vi "final_usrp_transceiver.vi"() -> ()   [LabVIEW 2014]
uses:
  <vilib>/vision/Image Controls.llb/IMAQ Image.ctl
  <vilib>/addons/Modulation/Digital/General/MT Generate Bits (Galois, PN Order).vi
  <vilib>/Analysis/2dsp.llb/Inverse Complex FFT.vi
  <vilib>/Analysis/2dsp.llb/Complex FFT.vi
  <vilib>/Analysis/5stat.llb/RMS (DBL).vi
  <vilib>/addons/Modulation/Digital/Support/Common/Validators/mod_Generate Bits Validate.vi
  <vilib>/addons/Modulation/Analog/support/mod_Set Error Source.vi
  var_stop.vi
  <vilib>/addons/Modulation/Digital/Support/Common/Validators/mod_Generate Filter Coefficients Validate.vi
  <vilib>/addons/Modulation/Digital/General/subVIs/mod_Generate Filter Coefficients.vi
  <vilib>/addons/Modulation/Digital/General/subVIs/mod_Generate Bits PN Sequence.vi
  <vilib>/addons/Modulation/Digital/General/MT Generate QAM System Parameters(M).vi
  <vilib>/addons/Modulation/Digital/General/MT Apply Pulse Shaping Filter (Generic).vi
  <instrlib>/niUSRP/niUSRP Write Tx Data (CDB Cluster).vi
  <vilib>/addons/Modulation/Digital/General/MT Apply Matched Filter (Generic).vi
  <vilib>/addons/Modulation/Digital/General/MT Align to Ideal Symbols (Generic).vi
  <vilib>/addons/Modulation/Digital/General/MT Map QAM Symbols to Bits.vi
  <instrlib>/niUSRP/niUSRP Fetch Rx Data (CDB Cluster).vi
  <vilib>/addons/Modulation/niDMT.lvlib
  <vilib>/Analysis/NI_AALPro.lvlib
panel:
  out "frame":T1(plugin-control)
  out "length 2":i32
  out "string":string
  out "number":u32
  out "pilot channel gain":dbl[](graph)
  out "pilot channel gain":dbl[](graph)
  out "PAPR":dbl
  in  "M-QAM (16)":i32=16
  out "TX buffer":i32
  out "RX buffer":i32
  out "avg energy":dbl
  in  "TX on":bool=TRUE
  in  "power scale":dbl format="%#_13g"
  out "acc recieved bits":i32
  out "acc error bits":i32
  out "Packet number":u8
  out "Packet bytes":u32
  out "past 20 error bits":i32[](array[numeric])
  in  "min_len":i32=200
  in  "Threshold":dbl=-61.0 format="%#_13g"
  out "Accumulated BER":dbl
  out "found packet":bool
  in  "total bits (128)":i32=1600 caption="bits per packet"
  in  "message carriers":i32=120
  out "RX  constellation map":cdb[](graph)
  in  "pilot carrier":i32=32
  in  "cyclic length":i32=64
  in  "FFT size":i32=256
  in  "filter length (symbols)":i32=8
  in  "filter parameter":dbl=0.35 format="%.2f"
  in  "samples per symbol (16)":i32=4
  in  "pulse shaping filter (none)":T2(ring)=enum."Root Raised Cos"
  in  "stop":bool
  in  "number of samples":i64=20000
  out "coerced carrier frequency":dbl format="%#_6p"
  out "coerced IQ rate":dbl format="%#_6p"
  in  "Clocking and Synchronization:Reference Frequency Source":string(combo)="Internal"
  in  "RX gain":dbl format="%#_6f"
  in  "TX gain":dbl format="%#_6f"
  in  "carrier frequency":dbl=915000000.0 format="%#_6p"
  in  "IQ rate":dbl=2000000.0 format="%#_6p"
  in  "RX device names":refnum<k15>="192.168.10.3"
  in  "TX device names":refnum<k15>="192.168.10.3"
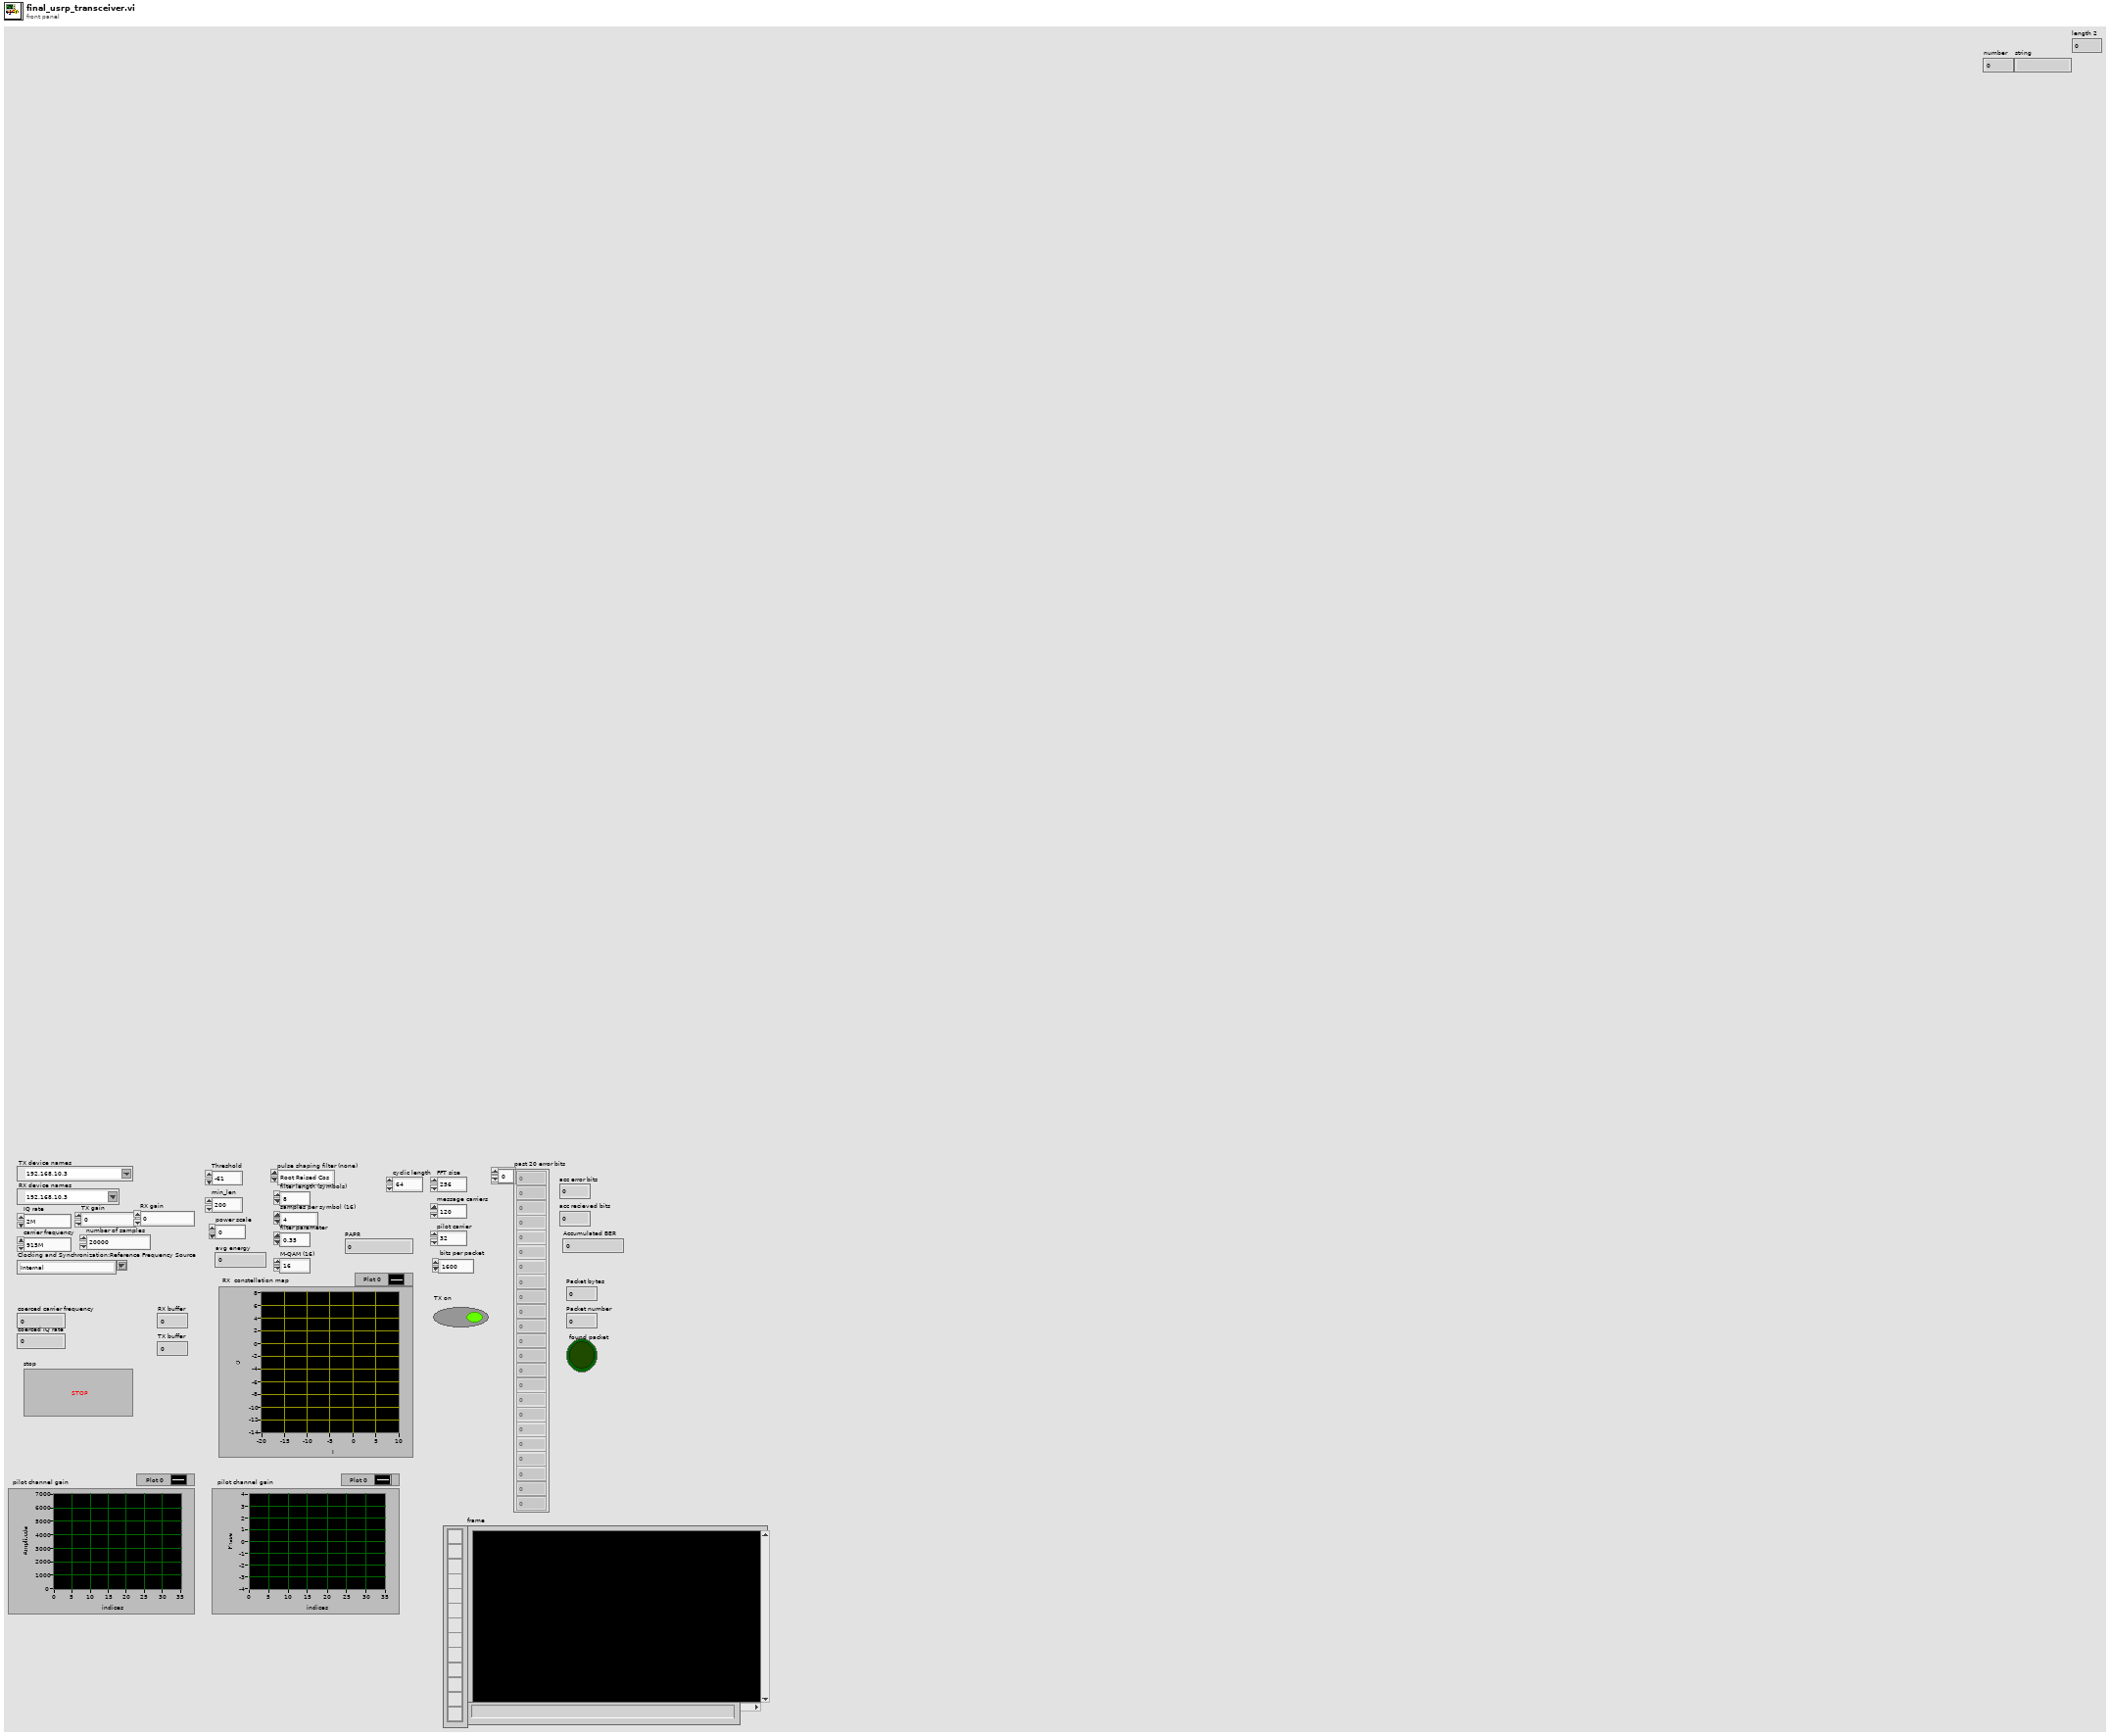
[diagram p1: front panel]
types:
  T1 = typedef "IMAQ Image.ctl" = refnum<image>
  T2 = enum16{"none", "Raised Cosine", "Root Raised Cos", "Gaussian"}
  T3 = enum16{"FSK", "PSK", "QAM", "MSK", "PAM", "ASK", "CPM"}
  T4 = cluster{"samples per symbol (16)":i32, "symbol map":cdb[]}
  T5 = typedef "niAMT.lvlib/Complex Data Waveform.ctl" = cluster{"t0":dbl, "dt":dbl, "Y":cdb[]}
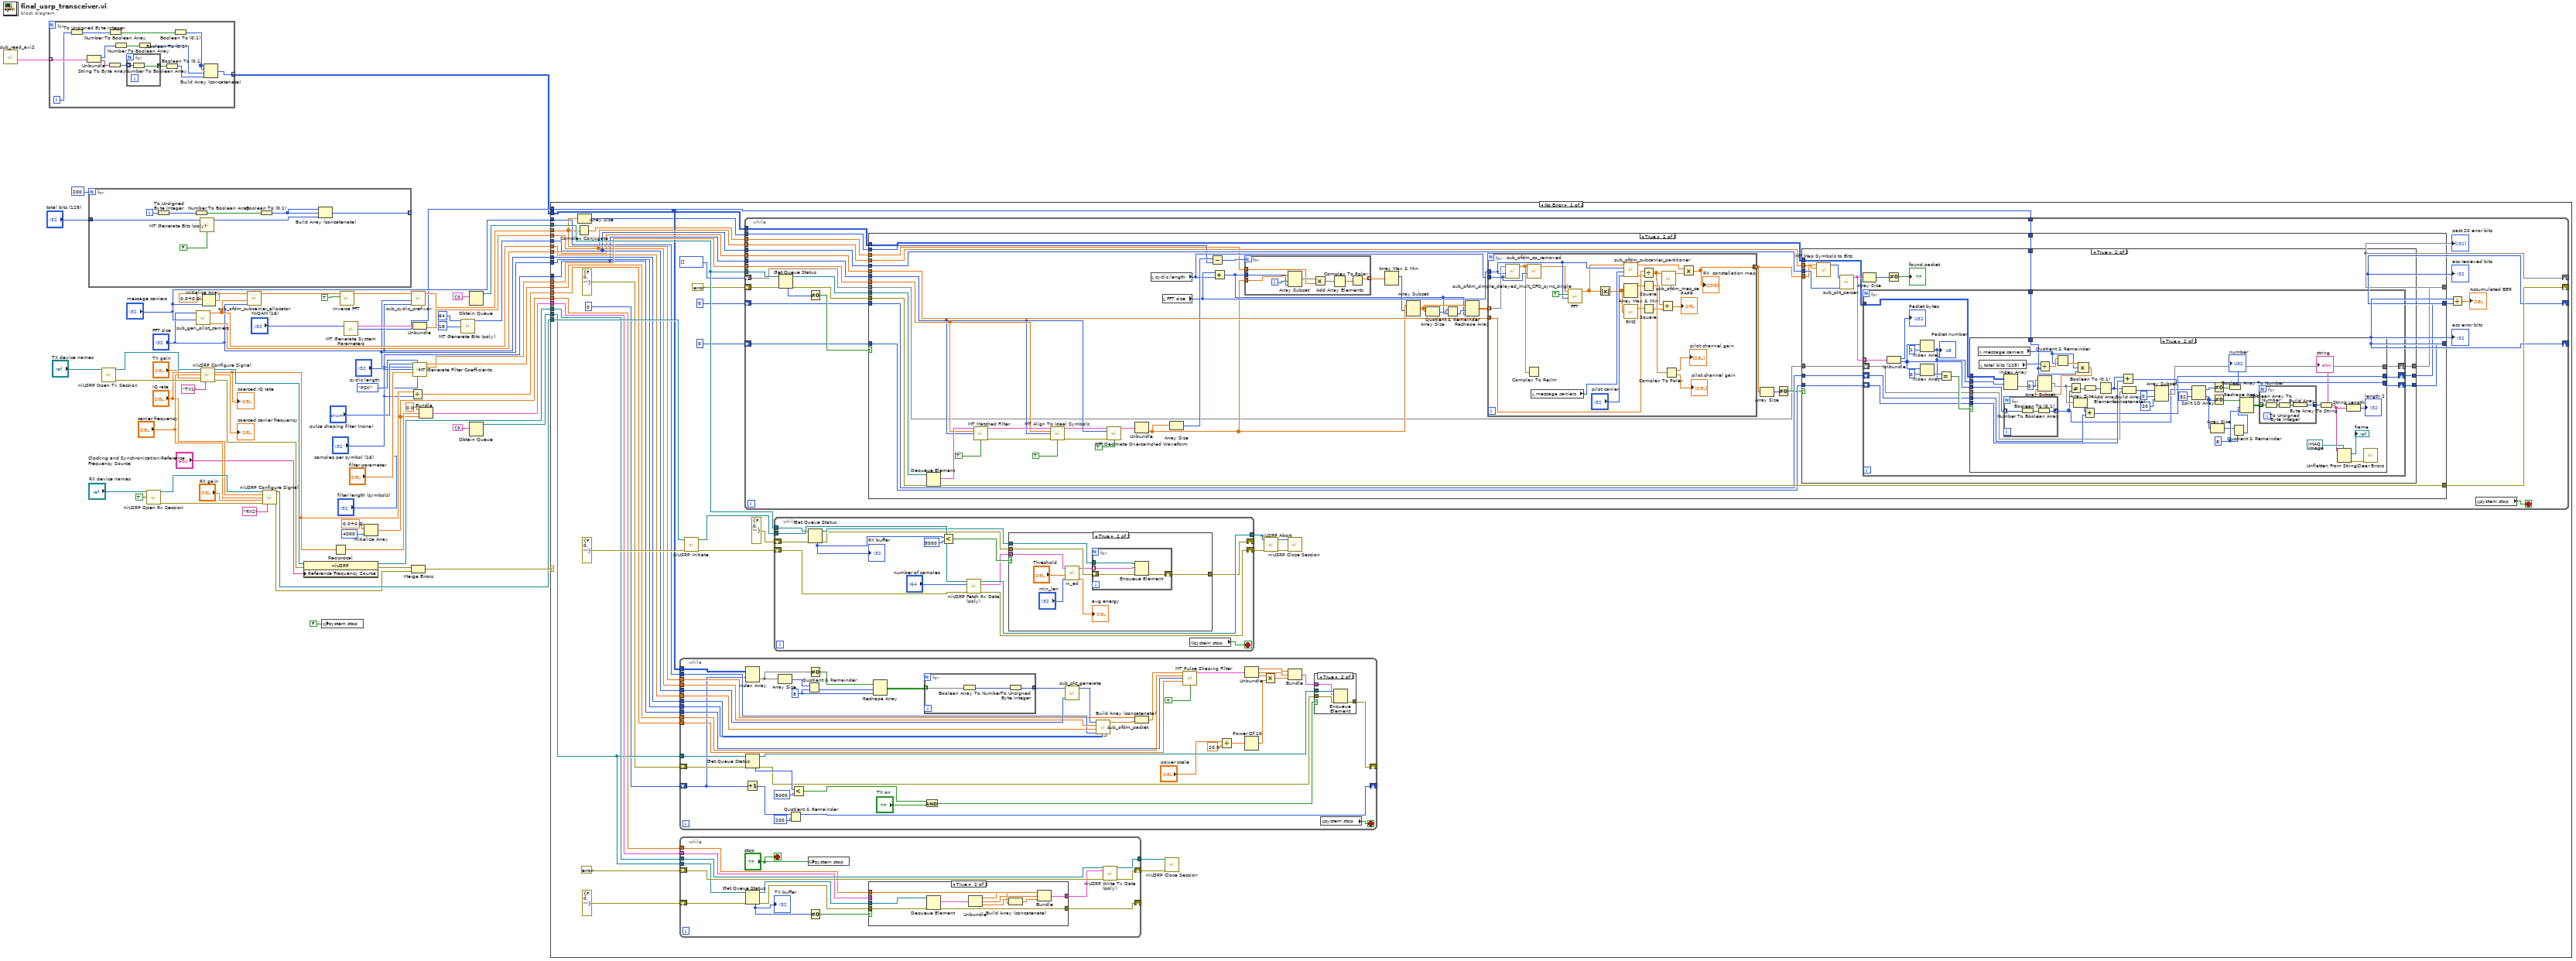
[diagram p0: block diagram]
diagram:
  n1 = call "sub_read_avi2.vi"() -> ("frames"=w2:cluster{i32, "Data String":string}[])  [unwired: 10 in, 1 out]
  n2 = for {
    tunnel: w2 -> [w70] mode=indexing
    tunnel: [w69] -> w1 mode=indexing
    i -> [w66]
    n3 = To Unsigned Byte Integer(number=w66) -> (unsigned 8bit integer=w68:u8)
    n4 = Unbundle(w70) -> (w75:i32, "Data String"=w71:string)
    n5 = String To Byte Array(string=w71) -> (unsigned byte array=w77:u8[])
    n6 = Number To Boolean Array(number=w68) -> (Boolean array=w67:bool[])
    n7 = Number To Boolean Array(number=w75) -> (Boolean array=w74:bool[])
    n8 = for {
      tunnel: w77 -> [w79] mode=indexing
      tunnel: [w78] -> w76 mode=concatenating
      n9 = Number To Boolean Array(number=w79) -> (Boolean array=w78:bool[])
    }
    n10 = Boolean To (0,1)(Boolean=w74) -> (0, 1=w72:i16[])
    n11 = Boolean To (0,1)(Boolean=w76) -> (0, 1=w73:i16[])
    n12 = Boolean To (0,1)(Boolean=w67) -> (0, 1=w65:i16[])
    n13 = Build Array (concatenate)(w65, w65, w72, w73) -> (w69:i16[])
  }
  n14 = for {
    N: 200 ("y") -> [_]
    tunnel: "total bits (128)" -> [w87]
    tunnel: [w80] -> _ mode=indexing
    i -> [w85]
    n15 = To Unsigned Byte Integer(number=w85) -> (unsigned 8bit integer=w84:u8)
    n16 = Number To Boolean Array(number=w84) -> (Boolean array=w83:bool[])
    n17 = call-poly <vilib>:"MT Generate Bits (poly).vi"("total bits (128)"=w87, "reset? (T)"=FALSE) -> ("output bit stream"=w81:i8[])  [unwired: 11 in, 2 out]
    n18 = Boolean To (0,1)(Boolean=w83) -> (0, 1=w82:i16[])
    n19 = Build Array (concatenate)(w82, w82, w81) -> (w80:i16[])
  }
  n20 = call <instrlib>:"niUSRP Open Tx Session.vi"("device names"="TX device names") -> ("session handle out"=w64:refnum<k15>, "error out"=w63:errorcluster)  [unwired: 13 in]
  n21 = call <instrlib>:"niUSRP Open Rx Session.vi"("device names"="RX device names", "reset"=TRUE) -> ("session handle out"=w60:refnum<k15>, "error out"=w59:errorcluster)  [unwired: 12 in]
  n22 = call "sub_gen_pilot_carriers.vi"("message carrier"="message carriers", "FFT size"="FFT size") -> ("RX pilot carriers"=w21:cdb[], "TX pilot carriers"=w17:cdb[])  [unwired: 8 in]
  n23 = call <instrlib>:"niUSRP Configure Signal.vi"("session handle"=w64, "IQ rate"="IQ rate", "carrier frequency"="carrier frequency", "gain"="TX gain", "error in (no error)"=w63, "active antenna"="TX1") -> ("session handle out"=w31:refnum<k15>, "coerced IQ rate"=w20:dbl, "coerced carrier frequency"=→"coerced carrier frequency":dbl, "error out"=w30:errorcluster)  [unwired: 5 in, 1 out]
  "coerced IQ rate" <- w20
  n24 = Initialize Array(cdb 0.0+0.0i, "message carriers") -> (w23:cdb[])
  n25 = call "sub_ofdm_subcarrier_allocator.vi"("fft size"="FFT size", "pilot symbol"=w17, "message symbol"=w23) -> ("OFDM symbol"=w16:cdb[])  [unwired: 8 in]
  n26 = call <instrlib>:"niUSRP Configure Signal.vi"("session handle"=w60, "IQ rate"="IQ rate", "carrier frequency"="carrier frequency", "gain"="RX gain", "error in (no error)"=w59, "active antenna"="RX2") -> ("session handle out"=w4:refnum<k15>, "error out"=w3:errorcluster)  [unwired: 5 in, 3 out]
  n27 = property class="niUSRP"(reference=w31, error in=w30, "Reference Frequency Source"="Clocking and Synchronization:Reference Frequency Source") -> (reference out=w45:refnum<k15>, error out=w50:errorcluster)
  n28 = global write "var_stop.vi" "system stop"(FALSE) -> ()
  n29 = Reciprocal(x=w20) -> (1/x=w40:dbl)
  n30 = call-poly <vilib>:"Inverse FFT.vi"("shift?"=TRUE, "FFT {X}"=w16) -> ("X"=w14:cdb[])  [unwired: 8 in, 1 out]
  n31 = call-poly <vilib>:"MT Generate System Parameters.vi"("M-QAM (16)"="M-QAM (16)") -> ("QAM system parameters"=w29:T4, "bits per symbol"=w6:i32)  [unwired: 12 in, 1 out]
  n32 = Initialize Array(cdb 0.0+0.0i, 4000 ("dimension size")) -> (w8:cdb[])
  n33 = Divide(x=w20, y="samples per symbol (16)") -> (x/y=w19:dbl)
  n34 = call "sub_cyclic_prefixer.vi"("FFT size"="FFT size", "CP length"="cyclic length", "time_samples"=w14) -> ("cp ofdm symbol"=w11:cdb[])  [unwired: 8 in]
  n35 = Merge Errors(w50, w3) -> (w49:errorcluster)
  n36 = Unbundle(w29) -> ("symbol map"=w28:cdb[])  [unwired: 1 out]
  n37 = call <vilib>:"MT Generate Filter Coefficients.vi"("pulse shaping filter (none)"="pulse shaping filter (none)", "modulation type"=T3."PSK", "pulse shaping samples per symbol (16)"="samples per symbol (16)", "matched samples per symbol (16)"="samples per symbol (16)", "filter parameter"="filter parameter", "filter length (symbols)"="filter length (symbols)") -> ("pulse shaping filter coefficients"=w34:dbl[], "matched filter coefficients"=w33:dbl[])  [unwired: 7 in, 1 out]
  n38 = Bundle(0.0, w40, w8) -> (w38:cluster{dbl, dbl, cdb[]})  [unwired: 1 in]
  n39 = call-poly <vilib>:"MT Generate Bits (poly).vi"("total bits (128)"=64, "PN sequence order (9)"=15) -> ("output bit stream"=w25:i8[])  [unwired: 11 in, 2 out]
  n40 = Obtain Queue(element data type=cluster{"t0":dbl, "dt":dbl, "Y":cdb[]} {"t0"=0.0, "dt"=0.0, "Y"=[]} ("data")) -> (queue out=w46:refnum<queue>)  [unwired: 4 in, 2 out]
  n41 = Obtain Queue(element data type=cluster{"t0":dbl, "dt":dbl, "Y":cdb[]} {"t0"=0.0, "dt"=0.0, "Y"=[]} ("data")) -> (queue out=w43:refnum<queue>)  [unwired: 4 in, 2 out]
  n42 = case shown="No Error" w49 {
    tunnel: w4 -> [w125 _]
    tunnel: w46 -> [w120 _]
    tunnel: w45 -> [w115 _]
    tunnel: w43 -> [w112 _]
    tunnel: w38 -> [w113 _]
    tunnel: w34 -> [w110 _]
    tunnel: w33 -> [w109 _]
    tunnel: "message carriers" -> [w106 _]
    tunnel: "FFT size" -> [w105 _]
    tunnel: w28 -> [w104 _]
    tunnel: w25 -> [w103 _]
    tunnel: w21 -> [w102 _]
    tunnel: w19 -> [w101 _]
    tunnel: "samples per symbol (16)" -> [w98 _]
    tunnel: w17 -> [w100 _]
    tunnel: "cyclic length" -> [w99 _]
    tunnel: w11 -> [w92 _]
    tunnel: w1 -> [w96 _]
    tunnel: w8 -> [w93 _]
    tunnel: w6 -> [w88 _]
    frame No Error {
      n43 = Complex Conjugate(1:w92) -> (0:w90:cdb[])
      n44 = Array Size(array=w92) -> (size(s)=w91:i32)
      n45 = while {
        tunnel: w112 -> [w167]
        shift-right: [w169] -> _
        shift-left: errorcluster {"status"=FALSE, "code"=0, "source"=""} ("error out") -> [w168]
        tunnel: w100 -> [w159]
        tunnel: w110 -> [w166]
        tunnel: w98 -> [w165]
        tunnel: w101 -> [w164]
        tunnel: w106 -> [w158]
        tunnel: w105 -> [w157]
        tunnel: w104 -> [w160]
        tunnel: w103 -> [w162]
        tunnel: w99 -> [w156]
        tunnel: w92 -> [w155]
        tunnel: w96 -> [w152]
        shift-right: [w148] -> _
        shift-left: 0 -> [w151]
        stop <- w174 stop-if-true
        w145 = 8 ("y")
        n46 = Increment(x=w151) -> (x+1=w150:i32)
        n47 = Index Array(array=w152, index (row)=w151) -> (element=w144:i16[])  [unwired: 1 in]
        n48 = Get Queue Status(queue=w167, error in (no error)=w168) -> (queue out=w171:refnum<queue>, error out=w170:errorcluster, # elements in queue=w173:i32)  [unwired: 1 in, 5 out]
        n49 = Array Size(array=w144) -> (size(s)=w147:i32)
        n50 = Quotient & Remainder(x=w150, y=200) -> (x-y*floor(x/y)=w148:i32)  [unwired: 1 out]
        n51 = Less?(x=w173, y=5000) -> (x < y?=w130:bool)
        n52 = Quotient & Remainder(x=w147, y=w145) -> (floor(x/y)=w146:i32)  [unwired: 1 out]
        n53 = Not Equal To 0?(x=w144) -> (x != 0?=w143:bool[])
        n54 = Reshape Array(w143, w146, w145) -> (w142:bool[][])
        n55 = for {
          tunnel: w142 -> [w177] mode=indexing
          tunnel: [w175] -> w141 mode=indexing
          n56 = Boolean Array To Number(Boolean array=w177) -> (number=w176:u32)
          n57 = To Unsigned Byte Integer(number=w176) -> (unsigned 8bit integer=w175:u8)
        }
        n58 = And(x=w130, y="TX on") -> (x .and. y?=w128:bool)
        n59 = call "sub_pkt_generate.vi"("accesscode (bit)"=w162, "byte stream"=w141) -> ("bit pkt"=w161:i16[])  [unwired: 9 in]
        n60 = call "sub_ofdm_packet.vi"("CP length"=w156, "FFT size"=w157, "message carriers"=w158, "pilot symbol"=w159, "symbol map"=w160, "packet"=w161) -> ("ofdm packet"=w154:cdb[])  [unwired: 5 in]
        n61 = Build Array (concatenate)(w155, w154) -> (w153:cdb[])
        n62 = call-poly <vilib>:"MT Pulse Shaping Filter.vi"("symbols"=w153, "pulse shaping filter coefficients"=w166, "samples per symbol (16)"=w165, "symbol rate (Hz)"=w164, "reset? (T)"=TRUE) -> ("output complex waveform"=w137:T5)  [unwired: 9 in, 1 out]
        n63 = Divide(x="power scale", y=20.0) -> (x/y=w138:dbl)
        n64 = Unbundle(w137) -> ("t0"=w132:dbl, "dt"=w133:dbl, "Y"=w136:cdb[])
        n65 = Power Of 10(x=w138) -> (10^x=w135:dbl)
        n66 = Multiply(x=w136, y=w135) -> (x*y=w134:cdb[])
        n67 = Bundle("t0"=w132, "dt"=w133, w134) -> (w131:cluster{"t0":dbl, "dt":dbl, cdb[]})  [unwired: 1 in]
        n68 = case shown="True" w128 {
          tunnel: w171 -> [_ w182]
          tunnel: w170 -> [w178 w181]
          tunnel: [w178 w180] -> w169
          tunnel: w131 -> [_ w179]
          frame False {
          }
          frame True {
            n69 = Enqueue Element(queue=w182, element=w179, error in (no error)=w181) -> (error out=w180:errorcluster)  [unwired: 1 in, 2 out]
          }
        }
        n70 = global read "var_stop.vi" "system stop"() -> (w174:bool)
      }
      n71 = while {
        tunnel: [w411] -> w118
        shift-right: [w410] -> w117
        shift-left: errorcluster {"status"=FALSE, "code"=0, "source"=""} ("error out") -> [w408]
        tunnel: w115 -> [w409]
        tunnel: w112 -> [w407]
        shift-right: [w401] -> _
        shift-left: errorcluster {"status"=FALSE, "code"=0, "source"=""} ("error out") -> [w406]
        tunnel: w113 -> [w400]
        tunnel: w93 -> [w399]
        stop <- "stop" stop-if-true
        n72 = Get Queue Status(queue=w407, error in (no error)=w406) -> (queue out=w403:refnum<queue>, error out=w404:errorcluster, # elements in queue=w405:i32)  [unwired: 1 in, 5 out]
        "TX buffer" <- w405
        n73 = global write "var_stop.vi" "system stop"("stop") -> ()
        n74 = Not Equal To 0?(x=w405) -> (x != 0?=w398:bool)
        n75 = case shown="True" w398 {
          tunnel: w404 -> [w414 w423]
          tunnel: w403 -> [_ w424]
          tunnel: [w413 w415] -> w402
          tunnel: [w414 w422] -> w401
          tunnel: w400 -> [w413 _]
          tunnel: w399 -> [_ w419]
          frame False {
          }
          frame True {
            n76 = Dequeue Element(queue=w424, error in (no error)=w423) -> (element=w421:cluster{"t0":dbl, "dt":dbl, "Y":cdb[]}, error out=w422:errorcluster)  [unwired: 1 in, 2 out]
            n77 = Unbundle(w421) -> ("t0"=w416:dbl, "dt"=w417:dbl, "Y"=w420:cdb[])
            n78 = Build Array (concatenate)(w420, w419) -> (w418:cdb[])
            n79 = Bundle("t0"=w416, "dt"=w417, w418) -> (w415:cluster{"t0":dbl, "dt":dbl, cdb[]})  [unwired: 1 in]
          }
        }
        n80 = call-poly <instrlib>:"niUSRP Write Tx Data (poly).vi"("session handle"=w409, "data"=w402, "error in (no error)"=w408) -> ("session handle out"=w411:refnum<k15>, "error out"=w410:errorcluster)  [unwired: 11 in]
      }
      n81 = call <instrlib>:"niUSRP Initiate.vi"("session handle"=w125, "error in (no error)"=errorcluster {"status"=FALSE, "code"=0, "source"=""}) -> ("session handle out"=w127:refnum<k15>, "error out"=w126:errorcluster)  [unwired: 12 in]
      n82 = while {
        tunnel: w120 -> [w201]
        shift-right: [w199] -> _
        shift-left: errorcluster {"status"=FALSE, "code"=0, "source"=""} ("error out") -> [w200]
        tunnel: w109 -> [w198]
        tunnel: w98 -> [w197]
        tunnel: w102 -> [w196]
        tunnel: w104 -> [w195]
        tunnel: w103 -> [w194]
        tunnel: w96 -> [w193]
        shift-right: [w189] -> _
        shift-left: 0 -> [w191]
        shift-right: [w190] -> _
        shift-left: 0 -> [w192]
        tunnel: w91 -> [w187]
        tunnel: w90 -> [w186]
        shift-right: [w184] -> _
        shift-left: i32[] [] -> [w185]
        tunnel: w88 -> [w183]
        stop <- w206 stop-if-true
        n83 = Get Queue Status(queue=w201, error in (no error)=w200) -> (queue out=w202:refnum<queue>, error out=w203:errorcluster, # elements in queue=w205:i32)  [unwired: 1 in, 5 out]
        n84 = Not Equal To 0?(x=w205) -> (x != 0?=w204:bool)
        n85 = case shown="True" w204 {
          tunnel: w203 -> [w210 w252]
          tunnel: w202 -> [_ w251]
          tunnel: [w210 w250] -> w199
          tunnel: w198 -> [_ w242]
          tunnel: w197 -> [_ w241]
          tunnel: w196 -> [_ w245]
          tunnel: w195 -> [_ w237]
          tunnel: w194 -> [_ w236]
          tunnel: w193 -> [_ w235]
          tunnel: w192 -> [w209 w234]
          tunnel: w191 -> [w208 w233]
          tunnel: [w209 w232] -> w190
          tunnel: [w208 w231] -> w189
          tunnel: w187 -> [_ w226]
          tunnel: w186 -> [_ w222]
          tunnel: w185 -> [w207 w213]
          tunnel: [w207 w212] -> w184
          tunnel: w183 -> [_ w211]
          frame False {
          }
          frame True {
            n86 = Dequeue Element(queue=w251, error in (no error)=w252) -> (element=w249:cluster{"t0":dbl, "dt":dbl, "Y":cdb[]}, error out=w250:errorcluster)  [unwired: 1 in, 2 out]
            n87 = call-poly <vilib>:"MT Matched Filter.vi"("input complex waveform"=w249, "matched filter coefficients"=w242, "samples per symbol (16)"=w241, "reset? (T)"=TRUE) -> ("output complex waveform"=w244:T5, "error out"=w243:errorcluster)  [unwired: 10 in]
            n88 = call-poly <vilib>:"MT Align To Ideal Symbols.vi"("input complex waveform"=w244, "matched filter coefficients"=w242, "samples per symbol (16)"=w241, "error in (no error)"=w243, "reset? (T)"=TRUE) -> ("output complex waveform"=w239:T5, "error out"=w238:errorcluster)  [unwired: 8 in, 1 out]
            n89 = call <vilib>:"MT Decimate Oversampled Waveform.vi"("input complex waveform"=w239, "decimation factor"=w241, "error in (no error)"=w238, "reset? (T)"=TRUE) -> ("output complex waveform"=w247:T5)  [unwired: 10 in, 1 out]
            n90 = Unbundle(w247) -> ("Y"=w220:cdb[])  [unwired: 2 out]
            n91 = local read "cyclic length"() -> (w223:i32)
            n92 = local read "FFT size"() -> (w224:i32)
            n93 = Array Size(array=w220) -> (size(s)=w227:i32)
            n94 = Subtract(x=w227, y=w226) -> (x-y=w225:i32)
            n95 = Add(x=w224, y=w223) -> (x+y=w215:i32)
            n96 = for {
              N: w225 -> [_]
              tunnel: w220 -> [w260]
              tunnel: w215 -> [w258]
              tunnel: w222 -> [w256]
              tunnel: [w253] -> w221 mode=indexing
              i -> [w259]
              n97 = Array Subset(array=w260, index=w259, length=w258) -> (w257:cdb[])
              n98 = Multiply(x=w257, y=w256) -> (x*y=w255:cdb[])
              n99 = Add Array Elements(numeric array=w255) -> (sum=w254:cdb)
              n100 = Complex To Polar(r * e^(i*theta)=w254) -> (r=w253:dbl)  [unwired: 1 out]
            }
            n101 = Array Max & Min(array=w221) -> (max index (indices)=w219:i32)  [unwired: 3 out]
            n102 = Array Subset(array=w220, index=w219) -> (w217:cdb[])  [unwired: 1 in]
            n103 = Array Size(array=w217) -> (size(s)=w218:i32)
            n104 = Quotient & Remainder(x=w218, y=w215) -> (floor(x/y)=w216:i32)  [unwired: 1 out]
            n105 = Reshape Array(w217, w216, w215) -> (w214:cdb[][])
            n106 = for {
              tunnel: w214 -> [w361] mode=indexing
              tunnel: w223 -> [w359]
              tunnel: w224 -> [w360]
              tunnel: [w366] -> w230 mode=concatenating
              tunnel: w245 -> [w363]
              n107 = call "sub_ofdm_simple_delayed_mult_CFO_sync_single.vi"("CP length"=w359, "FFT size"=w360, "time samples"=w361) -> ("sync ofdm symbol"=w350:cdb[])  [unwired: 8 in]
              n108 = call "sub_ofdm_cp_removed.vi"("CP length"=w359, "time ofdm symbol"=w350) -> ("cp removed ofdm symbol"=w351:cdb[])  [unwired: 9 in]
              n109 = Complex To Re/Im(x + iy=w350) -> ()  [unwired: 2 out]
              n110 = local read "message carriers"() -> (w365:i32)
              n111 = call-poly <vilib>:"FFT.vi"("FFT size"=w360, "shift?"=TRUE, "X"=w351) -> ("FFT {X}"=w358:cdb[])  [unwired: 7 in, 1 out]
              n112 = Absolute Value(x=w358) -> (abs(x)=w352:dbl[])
              n113 = call "sub_ofdm_subcarrier_partitioner.vi"("pilot carrier"="pilot carrier", "message carrier"=w365, "FFT size"=w360, "received symbol"=w358) -> ("pilot subcarriers"=w362:cdb[], "message subcarriers"=w364:cdb[])  [unwired: 6 in]
              n114 = Array Max & Min(array=w352) -> (max value=w357:dbl)  [unwired: 3 out]
              n115 = call-poly <vilib>:"RMS.vi"("X"=w352) -> ("rms value"=w355:dbl)  [unwired: 1 out]
              n116 = Divide(x=w363, y=w362) -> (x/y=w347:cdb[])
              n117 = Square(x=w357) -> (x^2=w356:dbl)
              n118 = Square(x=w355) -> (x^2=w354:dbl)
              n119 = Divide(x=w356, y=w354) -> (x/y=→"PAPR":dbl)
              n120 = call "sub_ofdm_mes_ce.vi"("ZF channel estimates"=w347) -> ("interpolated mes carrier CE"=w367:cdb[])  [unwired: 10 in]
              n121 = Complex To Polar(r * e^(i*theta)=w347) -> (r=→"pilot channel gain":dbl[], theta=→"pilot channel gain":dbl[])
              n122 = Multiply(x=w364, y=w367) -> (x*y=w366:cdb[])
              "RX  constellation map" <- w366
            }
            n123 = Array Size(array=w230) -> (size(s)=w229:i32)
            n124 = Not Equal To 0?(x=w229) -> (x != 0?=w228:bool)
            n125 = case shown="True" w228 {
              tunnel: w237 -> [_ w278]
              tunnel: w236 -> [_ w276]
              tunnel: w235 -> [_ w272]
              tunnel: w234 -> [w263 w271]
              tunnel: w233 -> [w262 w270]
              tunnel: [w263 w269] -> w232
              tunnel: [w262 w268] -> w231
              tunnel: w230 -> [_ w267]
              tunnel: w213 -> [w261 w266]
              tunnel: [w261 w265] -> w212
              tunnel: w211 -> [_ w264]
              frame False {
              }
              frame True {
                n126 = call-poly <vilib>:"MT Map Symbols to Bits.vi"("symbols"=w267, "symbol map"=w278) -> ("output bit stream"=w277:i8[])  [unwired: 12 in, 1 out]
                n127 = call "sub_pkt_parser.vi"("accesscode (bit)"=w276, "bitstream"=w277) -> ("parsed packet"=w273:cluster{"t":u32, "byte_array":u8[]}[])  [unwired: 9 in]
                n128 = Array Size(array=w273) -> (size(s)=w275:i32)
                n129 = for {
                  tunnel: w273 -> [w294] mode=indexing
                  tunnel: w272 -> [w288]
                  shift-right: [w285] -> w269
                  shift-left: w271 -> [w286]
                  shift-right: [w283] -> w268
                  shift-left: w270 -> [w284]
                  shift-right: [w281] -> w265
                  shift-left: w266 -> [w282]
                  tunnel: w264 -> [w279]
                  n130 = Unbundle(w294) -> ("t"=→"Packet bytes":u32, "byte_array"=w289:u8[])
                  n131 = Index Array(array=w289, index=1) -> (element=w287:u8)
                  "Packet number" <- w287
                  n132 = Index Array(array=w289, index=0) -> (element=w291:u8)
                  n133 = Equal?(x=w291, y=w287) -> (x = y?=w290:bool)
                  n134 = case shown="True" w290 {
                    tunnel: w289 -> [_ w325]
                    tunnel: w288 -> [_ w339]
                    tunnel: w287 -> [_ w338]
                    tunnel: w286 -> [w297 w335]
                    tunnel: [w297 w334] -> w285
                    tunnel: w284 -> [w296 w333]
                    tunnel: [w296 w332] -> w283
                    tunnel: w282 -> [w295 w331]
                    tunnel: [w295 w326] -> w281
                    tunnel: w279 -> [_ w320]
                    frame False {
                    }
                    frame True {
                      w310 = 8 ("y")
                      n135 = local read "message carriers"() -> (w321:i32)
                      n136 = local read "total bits (128)"() -> (w324:i32)
                      n137 = Index Array(array=w339, index (row)=w338) -> (element=w319:i16[])  [unwired: 1 in]
                      n138 = for {
                        tunnel: w325 -> [w346] mode=indexing
                        tunnel: [w344] -> w302 mode=concatenating
                        n139 = Number To Boolean Array(number=w346) -> (Boolean array=w345:bool[])
                        n140 = Boolean To (0,1)(Boolean=w345) -> (0, 1=w344:i16[])
                      }
                      n141 = Divide(x=w324, y=w320) -> (x/y=w323:dbl)
                      n142 = Quotient & Remainder(x=w323, y=w321) -> (floor(x/y)=w322:dbl)  [unwired: 1 out]
                      n143 = Compound Arithmetic op=MULTIPLY(w322, w321, w320) -> (w317:dbl)
                      n144 = Array Subset(array=w319, index=0, length=w317) -> (w316:i16[])
                      n145 = Not Equal?(x=w316, y=w302) -> (x != y?=w337:bool[])
                      n146 = Array Size(array=w316) -> (size(s)=w315:i32)
                      n147 = Boolean To (0,1)(Boolean=w337) -> (0, 1=w336:i16[])
                      n148 = Add(x=w315, y=w333) -> (x+y=w332:i32)
                      n149 = Add Array Elements(numeric array=w336) -> (sum=w330:i16)
                      n150 = Add(x=w330, y=w335) -> (x+y=w334:i32)
                      n151 = Build Array (concatenate)(w330, w331) -> (w329:i32[])
                      n152 = Array Subset(array=w329, index=0, length=20) -> (w326:i32[])
                      n153 = Split 1D Array(array=w302, index=32) -> (first subarray=w304:i16[], second subarray=w307:i16[])
                      n154 = Array Size(array=w307) -> (size(s)=w308:i32)
                      n155 = Not Equal To 0?(x=w304) -> (x != 0?=w305:bool[])
                      n156 = Not Equal To 0?(x=w307) -> (x != 0?=w306:bool[])
                      n157 = Boolean Array To Number(Boolean array=w305) -> (number=→"number":u32)
                      n158 = Quotient & Remainder(x=w308, y=w310) -> (floor(x/y)=w309:i32)  [unwired: 1 out]
                      n159 = Reshape Array(w306, w309, w310) -> (w311:bool[][])
                      n160 = for {
                        tunnel: w311 -> [w343] mode=indexing
                        tunnel: [w341] -> w312 mode=concatenating
                        n161 = Boolean Array To Number(Boolean array=w343) -> (number=w342:u32)
                        n162 = To Unsigned Byte Integer(number=w342) -> (unsigned 8bit integer=w340:u8)
                        n163 = Build Array(w340) -> (w341:u8[])
                      }
                      n164 = Byte Array To String(unsigned byte array=w312) -> (string=w299:string)
                      "string" <- w299
                      n165 = Unflatten From String(type=T1 refnum ("frame 2"), binary string=w299) -> (value=→"frame":T1, error out=w298:errorcluster)  [unwired: 3 in, 1 out]
                      n166 = String Length(string=w299) -> (length=→"length 2":i32)
                      n167 = call <vilib>:"Clear Errors.vi"("error in (no error)"=w298) -> ()  [unwired: 5 in, 2 out]
                    }
                  }
                }
                n168 = Not Equal To 0?(x=w275) -> (x != 0?=→"found packet":bool)
              }
            }
          }
        }
        "past 20 error bits" <- w184
        "acc error bits" <- w190
        "acc recieved bits" <- w189
        n169 = Divide(x=w190, y=w189) -> (x/y=→"Accumulated BER":dbl)
        n170 = global read "var_stop.vi" "system stop"() -> (w206:bool)
      }
      n171 = while {
        tunnel: w127 -> [w384]
        shift-right: [w377] -> w122
        shift-left: w126 -> [w383]
        tunnel: [w378] -> w123
        tunnel: w120 -> [w374]
        shift-right: [w372] -> _
        shift-left: errorcluster {"status"=FALSE, "code"=0, "source"=""} ("error out") -> [w371]
        stop <- w370 stop-if-true
        n172 = Get Queue Status(queue=w374, error in (no error)=w371) -> (queue out=w375:refnum<queue>, error out=w373:errorcluster, # elements in queue=w381:i32)  [unwired: 1 in, 5 out]
        "RX buffer" <- w381
        n173 = Less?(x=w381, y=5000) -> (x < y?=w379:bool)
        n174 = call-poly <instrlib>:"niUSRP Fetch Rx Data (poly).vi"("session handle"=w384, "number of samples"="number of samples", "error in (no error)"=w383) -> ("session handle out"=w378:refnum<k15>, "data"=w376:cluster{"t0":dbl, "dt":dbl, "Y":cdb[]}, "error out"=w377:errorcluster)  [unwired: 9 in, 1 out]
        n175 = case shown="True" w379 {
          tunnel: w376 -> [_ w390]
          tunnel: w375 -> [_ w391]
          tunnel: w373 -> [w385 w393]
          tunnel: [w385 w392] -> w372
          frame False {
          }
          frame True {
            n176 = call "rx_ed.vi"("min_len"="min_len", "Threshold"="Threshold", "Wavefrom"=w390) -> ("avg energy"=→"avg energy":dbl, "extract wav"=w387:cluster{"t0":dbl, "dt":dbl, cdb[]}[])  [unwired: 7 in]
            n177 = for {
              tunnel: w391 -> [w395]
              shift-right: [w396] -> w392
              shift-left: w393 -> [w397]
              tunnel: w387 -> [w394] mode=indexing
              n178 = Enqueue Element(queue=w395, element=w394, error in (no error)=w397) -> (error out=w396:errorcluster)  [unwired: 1 in, 2 out]
            }
          }
        }
        n179 = global read "var_stop.vi" "system stop"() -> (w370:bool)
      }
      n180 = call <instrlib>:"niUSRP Close Session.vi"("session handle"=w118, "error in (no error)"=w117) -> ()  [unwired: 13 in, 1 out]
      n181 = call <instrlib>:"niUSRP Abort.vi"("session handle"=w123, "error in (no error)"=w122) -> ("session handle out"=w108:refnum<k15>, "error out"=w107:errorcluster)  [unwired: 12 in]
      n182 = call <instrlib>:"niUSRP Close Session.vi"("session handle"=w108, "error in (no error)"=w107) -> ()  [unwired: 13 in, 1 out]
    }
    frame Error {
    }
  }
